vi "convertPercentageToU16Bits.vi"(8 "error in (no error)":errorcluster, 10 "Percentage (%)":dbl=2.0 min=0.0 max=100.0, 11 "Model in":refnum<class "Model.lvclass">) -> (0 "error out":errorcluster, 2 "u16Equivalent":u16=2 min=1 max=4, 3 "Model out":refnum<class "Model.lvclass">)   [LabVIEW 2015, in "Model.lvclass"]
uses:
  Model.lvclass
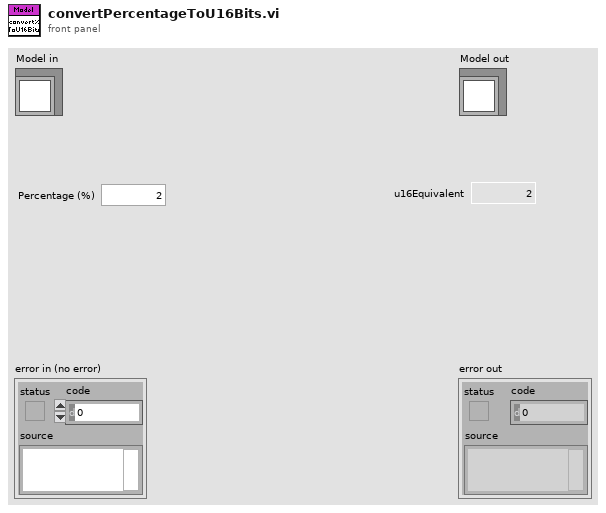
[diagram p1: front panel]
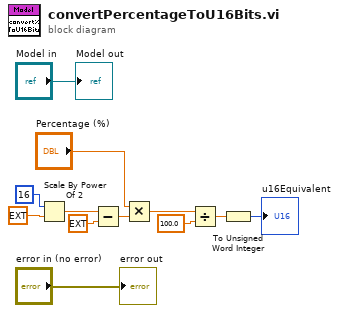
[diagram p0: block diagram]
diagram:
  n1 = Scale By Power Of 2(n=i16 16, x=ext 1.0) -> (x*2^n=w8:ext)
  n2 = Subtract(x=w8, y=ext 1.0) -> (x-y=w6:ext)
  n3 = Multiply(x="Percentage (%)", y=w6) -> (x*y=w3:ext)
  n4 = Divide(x=w3, y=100.0) -> (x/y=w1:ext)
  n5 = To Unsigned Word Integer(number=w1) -> (unsigned 16bit integer=→"u16Equivalent":u16)
  "error out" <- "error in (no error)"
  "Model out" <- "Model in"
